vi "Drive Direction.vi"(8 "error in":errorcluster, 9 "Velocity (mm/s)":i16, 10 "iRobot Drive Direction":T1=32768 items=["Straight"=32768, "Clockwise"=65535, "Counter-Clockwise"=1], 11 "UART port in":T2) -> (0 "error out":errorcluster, 3 "UART port out":T2)   [LabVIEW 2013]
doc: "Drive the robot straight, clockwise, or counter-clockwise.\n\nThis VI writes to, but does not read from, the serial port."
uses:
  Advanced/UART/iRobot UART Port Type.ctl
  Drive Direction.ctl
  Advanced/Command/OpCode.ctl
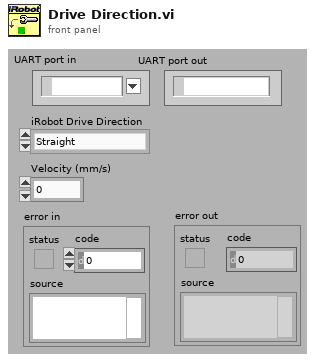
[diagram p1: front panel]
types:
  T1 = typedef "Drive Direction.ctl" = u16
  T2 = typedef "iRobot UART Port Type.ctl" = refnum<visa-resource-name>
  T3 = typedef "OpCode.ctl" = u8
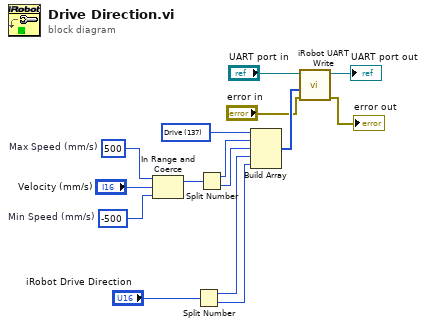
[diagram p0: block diagram]
diagram:
  w13 = i16 -500  # Min Speed (mm/s)
  w14 = i16 500  # Max Speed (mm/s)
  w7 = T3 137 items=["Start"=128, "Baud"=129, "Control"=130, "Safe"=131, "Full"=132, "Demo"=136, "Demo - Cover"=135, "Demo - Cover and Dock"=143, "Demo - Spot"=134, "Drive"=137, "Drive Direct"=145, "LEDs"=139, "Digital Outputs"=147, "PWM Low Side Drivers"=144, "Low Side Drivers"=138, "Send IR"=151, "Song"=140, "Play Song"=141, "Sensors"=142, "Query List"=149, "Stream"=148, "Pause/Resume Stream"=150, "Script"=152, "Play Script"=153, "Show Script"=154, "Wait Time"=155, "Wait Distance"=156, "Wait Angle"=157, "Wait Event"=158] ("OpCode")
  n1 = In Range and Coerce(upper limit=w14, x="Velocity (mm/s)", lower limit=w13) -> (coerced(x)=w12:i16)  [unwired: 1 out]
  n2 = Split Number(x="iRobot Drive Direction") -> (hi(x)=w9:u8, lo(x)=w8:u8)
  n3 = Split Number(x=w12) -> (hi(x)=w11:u8, lo(x)=w10:u8)
  n4 = Build Array(w7, w11, w10, w9, w8) -> (w6:T3[])
  n5 = call "iRobot UART Write.vi"("error in"="error in", "data"=w6, "UART port in"="UART port in") -> ("error out"=→"error out":errorcluster, "UART port out"=→"UART port out":T2)  [unwired: 7 in]
